vi "WinCI Has Project Open.vi"(8 "error in (no error)":errorcluster) -> (0 "error out":errorcluster, 2 "project open?":bool)   [LabVIEW 2020, in "NI_SCC_WinCI.lvlib"]
uses:
  <vilib>/SourceControl/Providers/WinCI/NI_SCC_WinCI.lvlib
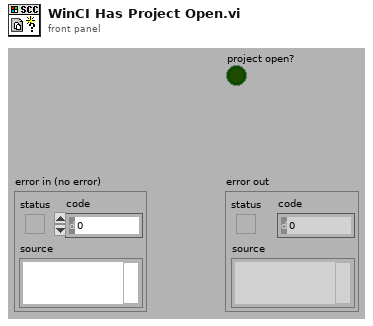
[diagram p1: front panel]
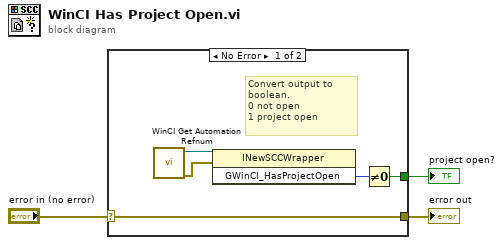
[diagram p0: block diagram]
diagram:
  n1 = case shown="No Error" "error in (no error)" {
    selector: "error in (no error)" -> [w7 w9]
    tunnel: [w7 w9] -> w2
    tunnel: [w8 _] -> w1
    frame No Error {
      # "Convert output to boolean.\n0 not open\n1 project open"
      n2 = call <vilib>:"WinCI Get Automation Refnum.vi"() -> ("error out"=w5:errorcluster, "automation refnum"=w4:refnum<k7>)  [unwired: 10 out]
      n3 = invoke class="INewSCCWrapper" method="GWinCI_HasProjectOpen"(reference=w4, error in=w5) -> ("GWinCI_HasProjectOpen"=w6:i32)  [unwired: 1 in, 2 out]
      n4 = Not Equal To 0?(x=w6) -> (x != 0?=w8:bool)
    }
    frame Error {
    }
  }
  "error out" <- w2
  "project open?" <- w1
